vi "Cannon Get.vi"(2 "Shoot!":T1) -> ()   [LabVIEW 2013]
uses:
  <vilib>/Rock Robotics/WPI/Solenoid/WPI_SolenoidValue.ctl
  Cannon Global Data.vi
panel:
  in  "Reset Gyro?":bool
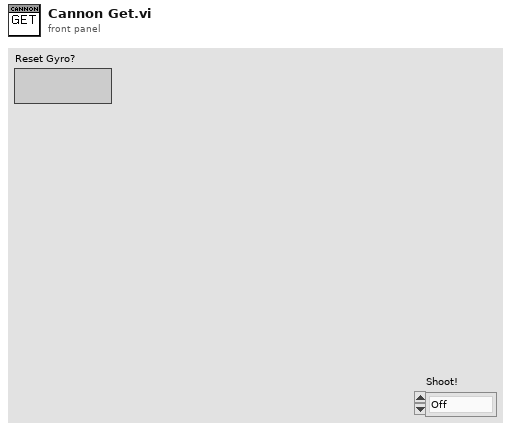
[diagram p1: front panel]
types:
  T1 = typedef "WPI_SolenoidValue.ctl" = enum16{"Off", "On", "Forward", "Reverse"}
  T2 = cluster{"MS":bool, "Shoot!":T1, "Angle":dbl, "Reset Gyro?":bool}
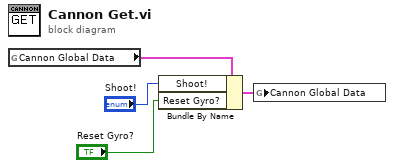
[diagram p0: block diagram]
diagram:
  n1 = global read "Cannon Global Data.vi" "Cannon Global Data"() -> (w3:T2)
  n2 = Bundle By Name(cluster=w3, "Shoot!"="Shoot!", "Reset Gyro?"="Reset Gyro?") -> (w2:T2)
  n3 = global write "Cannon Global Data.vi" "Cannon Global Data"(w2) -> ()
